vi "HOST sample code.vi"() -> ()   [LabVIEW 2020]
uses:
  <vilib>/Platform/TimedLoop/XDataNode/timing_clust.ctl
  <vilib>/Platform/TimedLoop/XDataNode/nitl_modes.ctl
  <vilib>/Platform/TimedLoop/XDataNode/wakeup.ctl
  <vilib>/Platform/TimedLoop/XDataNode/XDataNode.xnode
  <vilib>/Platform/TimedLoop/XDataNode/XDNodeRunTimeDep.lvlib
panel:
  out "Status word":u16
  in  "Sine test":bool caption="空白按钮"
  in  "Message ID":u32
  in  "descend":bool caption="空白按钮"
  in  "run":bool caption="空白按钮"
  in  "neutral":bool caption="空白按钮"
  in  "host ip":string="127.0.0.1"
  in  "base ip":string="127.0.0.1"
  in  "Command word":u16
  out "sway/surge/heave":T1(graph)
  out "pitch/roll/yaw":T2(graph)
  out "Stroke1..6":T3(graph)
  out "DataToHOST":T4 {"actuator6_pos" format="%#.2f"; "actuator5_pos" format="%#.2f"; "actuator4_pos" format="%#.2f"; "actuator3_pos" format="%#.2f"; "actuator2_pos" format="%#.2f"; "actuator1_pos" format="%#.2f"; "driver6 torque" format="%#.2f"; "driver5 torque" format="%#.2f"; "driver4 torque" format="%#.2f"; "driver3 torque" format="%#.2f"; "driver2 torque" format="%#.2f"; "driver1 torque" format="%#.2f"; "errorCode6(hex)" format="%x"; "errorCode5(hex)" format="%x"; "errorCode4(hex)" format="%x"; "errorCode3(hex)" format="%x"; "errorCode2(hex)" format="%x"; "errorCode1(hex)" format="%x"; "Heave actual" format="%#.2f"; "Surge actual" format="%#.2f"; "Sway actual" format="%#.2f"; "Yaw actual" format="%#.2f"; "Roll actual" format="%#.2f"; "Pitch actual" format="%#.2f"; "IO word" format="%x"}
  in  "host port":u16=10010
  in  "base port":u16=10000
  out "DataToDOF":T5={"Packet lenght"=48, "sequence count"=0, "Reserved"=0, "Message ID"=0, "Command word"=0, "Playback file ID"=0, "SubCmd"=0, "Reserved3"=0, "Reserved4"=0, "Reserved5"=0, "PITCH"=0.0, "ROLL"=0.0, "YAW"=0.0, "SWAY"=0.0, "SURGE"=0.0, "HEAVE"=0.0, "var11"=0.0, "var12"=0.0, "var13"=0.0, "var14"=0.0, "var15"=0.0, "var16"=0.0, "var21"=0.0, "var22"=0.0, "var23"=0.0, "var24"=0.0, "var25"=0.0, "var26"=0.0, "var31"=0.0, "var32"=0.0, "var33"=0.0, "var34"=0.0, "var35"=0.0, "var36"=0.0} {"Reserved5" format="%x"; "Reserved4" format="%x"; "Reserved3" format="%x"}
  in  "停止":bool
  # "概述：演示使用UDP通讯控制运动模拟器并显示其状态。\n操作步骤：\n1.网络链接运动模拟器，设置好IP和端口；\n2.运行VI，点击界面按钮，控制模拟器动作；\n3.单击停止 停止VI运行。"
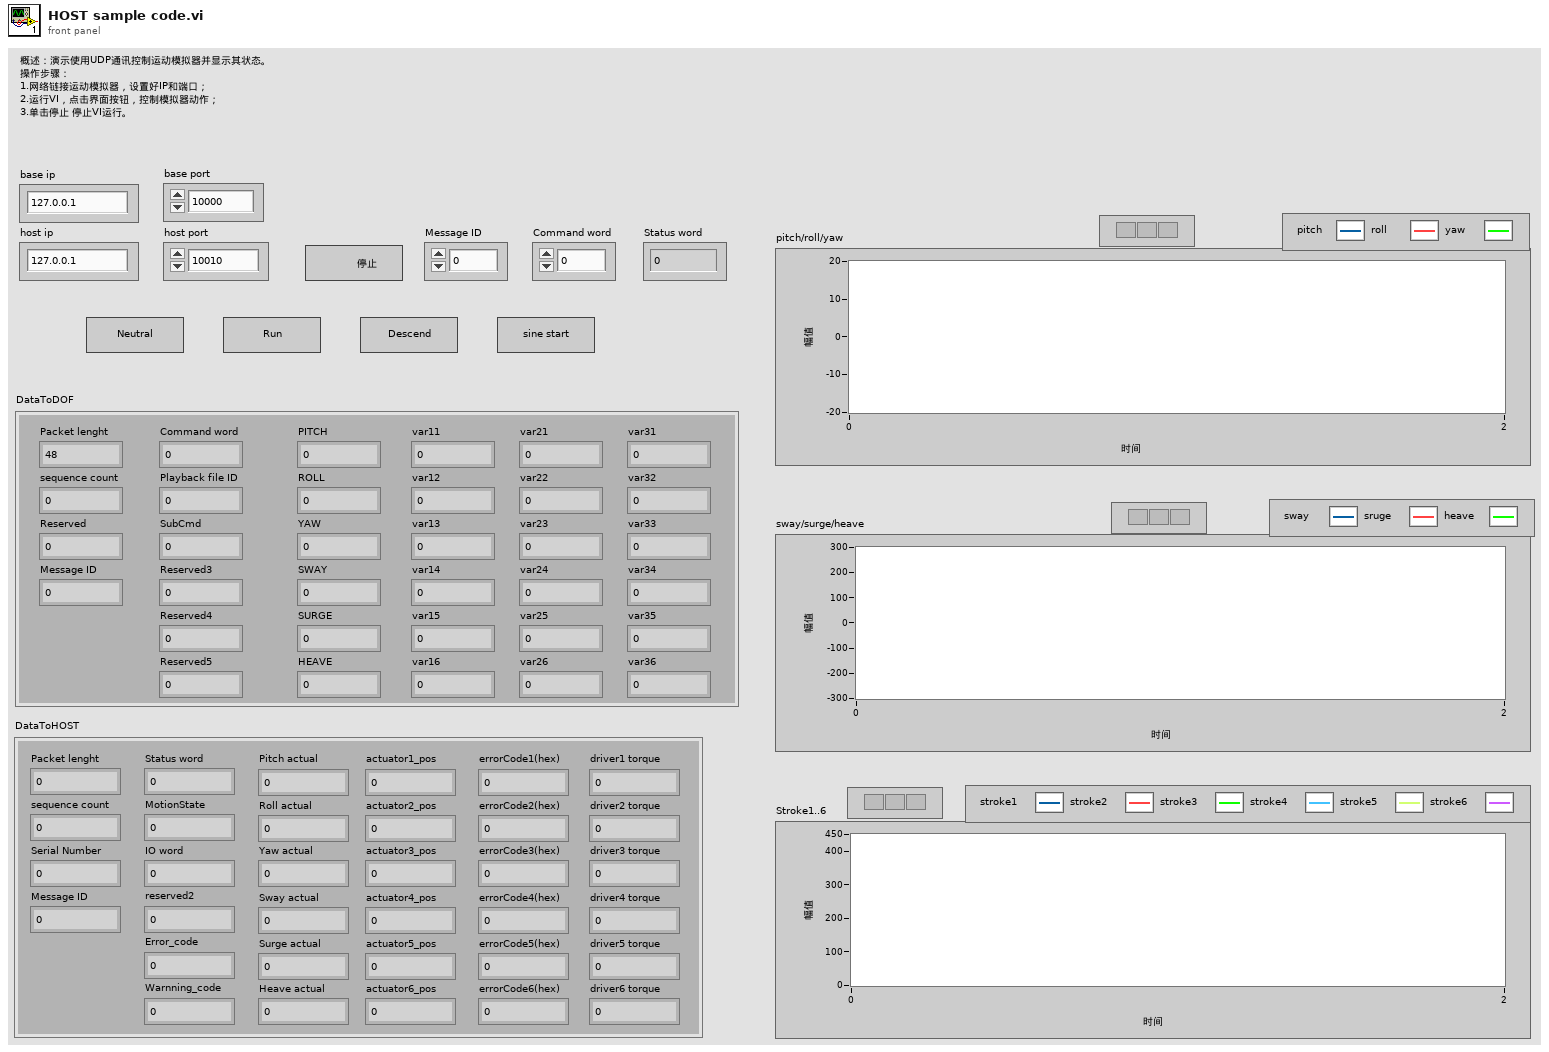
[diagram p1: front panel]
types:
  T1 = cluster{"Sway actual ":sgl, "Surge actual ":sgl, "Heave actual ":sgl}
  T2 = cluster{"Pitch actual ":sgl, "Roll actual ":sgl, "Yaw actual ":sgl}
  T3 = cluster{"actuator1_pos":sgl, "actuator2_pos":sgl, "actuator3_pos":sgl, "actuator4_pos":sgl, "actuator5_pos":sgl, "actuator6_pos":sgl}
  T4 = cluster{"Packet lenght":u32, "sequence count":u32, "Serial Number":u32, "Message ID":u32, "Status word":u16, "MotionState":u16, "IO word":u16, "reserved2":u16, "Error_code":u32, "Warnning_code":u32, "Pitch actual ":sgl, "Roll actual ":sgl, "Yaw actual ":sgl, "Sway actual ":sgl, "Surge actual ":sgl, "Heave actual ":sgl, "actuator1_pos":sgl, "actuator2_pos":sgl, "actuator3_pos":sgl, "actuator4_pos":sgl, "actuator5_pos":sgl, "actuator6_pos":sgl, "errorCode1(hex)":u32, "errorCode2(hex)":u32, "errorCode3(hex)":u32, "errorCode4(hex)":u32, "errorCode5(hex)":u32, "errorCode6(hex)":u32, "driver1 torque":sgl, "driver2 torque":sgl, "driver3 torque":sgl, "driver4 torque":sgl, "driver5 torque":sgl, "driver6 torque":sgl}
  T5 = cluster{"Packet lenght":u32, "sequence count":u32, "Reserved":u32, "Message ID":u32, "Command word":u16, "Playback file ID":u16, "SubCmd":u16, "Reserved3":u16, "Reserved4":u32, "Reserved5":u32, "PITCH":sgl, "ROLL":sgl, "YAW":sgl, "SWAY":sgl, "SURGE":sgl, "HEAVE":sgl, "var11":sgl, "var12":sgl, "var13":sgl, "var14":sgl, "var15":sgl, "var16":sgl, "var21":sgl, "var22":sgl, "var23":sgl, "var24":sgl, "var25":sgl, "var26":sgl, "var31":sgl, "var32":sgl, "var33":sgl, "var34":sgl, "var35":sgl, "var36":sgl}
  T6 = typedef "XDNodeRunTimeDep.lvlib/timing_clust.ctl" = cluster{"Expected End [f-1]":u64, "Actual End [f-1]":u64, "Finished Late? [f-1]":bool, "Expected End [i-1]":u64, "Actual End [i-1]":u64, "Finished Late? [i-1]":bool, "Expected Start [i]":u64, "Actual Start [i]":u64, "Expected Start [f]":u64, "Actual Start [f]":u64, "Source Name":string, "Structure Name":string, "Period":i64, "Deadline":i64, "Offset":i64, "Start":i64, "Priority":i32, "Timeout":i32, "Mode":T7, "Wakeup Reason":T8, "Error":errorcluster, "Source Type":string, "Secondary Source Type":string, "Global End Time":u64, "Global Start Time":u64, "Frame Duration":u64, "Iteration Duration":u64, "Assigned CPU":i32, "I/O Scan Engine Mode":u32}
  T7 = typedef "XDNodeRunTimeDep.lvlib/nitl_modes.ctl" = enum32{"No Change", "Process missed periods, maintain original phase", "Discard missed periods, maintain original phase", "Process missed periods, ignore original phase", "Discard missed periods, ignore original phase"}
  T8 = typedef "XDNodeRunTimeDep.lvlib/wakeup.ctl" = enum32{"Normal", "Aborted", "Asynchronous wakeup", "Timing source error", "Timed loop error", "Timeout"}
  T9 = cluster{"Packet lenght":u32, "sequence count":u32, "Reserved":u32, "Message ID":u32, "Status word":u16, "MotionState":u16, "IO word":u16, "reserved2":u16, "Error_code":u32, "Warnning_code":u32, "Pitch actual ":sgl, "Roll actual ":sgl, "Yaw actual ":sgl, "Sway actual ":sgl, "Surge actual ":sgl, "Heave actual ":sgl, "actuator1_pos":sgl, "actuator2_pos":sgl, "actuator3_pos":sgl, "actuator4_pos":sgl, "actuator5_pos":sgl, "actuator6_pos":sgl, "errorCode1":u32, "errorCode2":u32, "errorCode3":u32, "errorCode4":u32, "errorCode5":u32, "errorCode6":u32, "driver1 torque":sgl, "driver2 torque":sgl, "driver3 torque":sgl, "driver4 torque":sgl, "driver5 torque":sgl, "driver6 torque":sgl}
  T10 = enum16{"big-endian, network order", "native, host order", "little-endian"}
  T11 = cluster{"Packet lenght":u32, "sequence count":u32, "Reserved":u32, "Message ID":u32, "Command word":u16, "Playback file ID":u16, "Rserved2":u16, "Reserved3":u16, "Reserved4":u32, "Reserved5":u32, "PITCH":sgl, "ROLL":sgl, "YAW":sgl, "SWAY":sgl, "SURGE":sgl, "HEAVE":sgl, "var11":sgl, "var12":sgl, "var13":sgl, "var14":sgl, "var15":sgl, "var16":sgl, "var21":sgl, "var22":sgl, "var23":sgl, "var24":sgl, "var25":sgl, "var26":sgl, "var31":sgl, "var32":sgl, "var33":sgl, "var34":sgl, "var35":sgl, "var36":sgl}
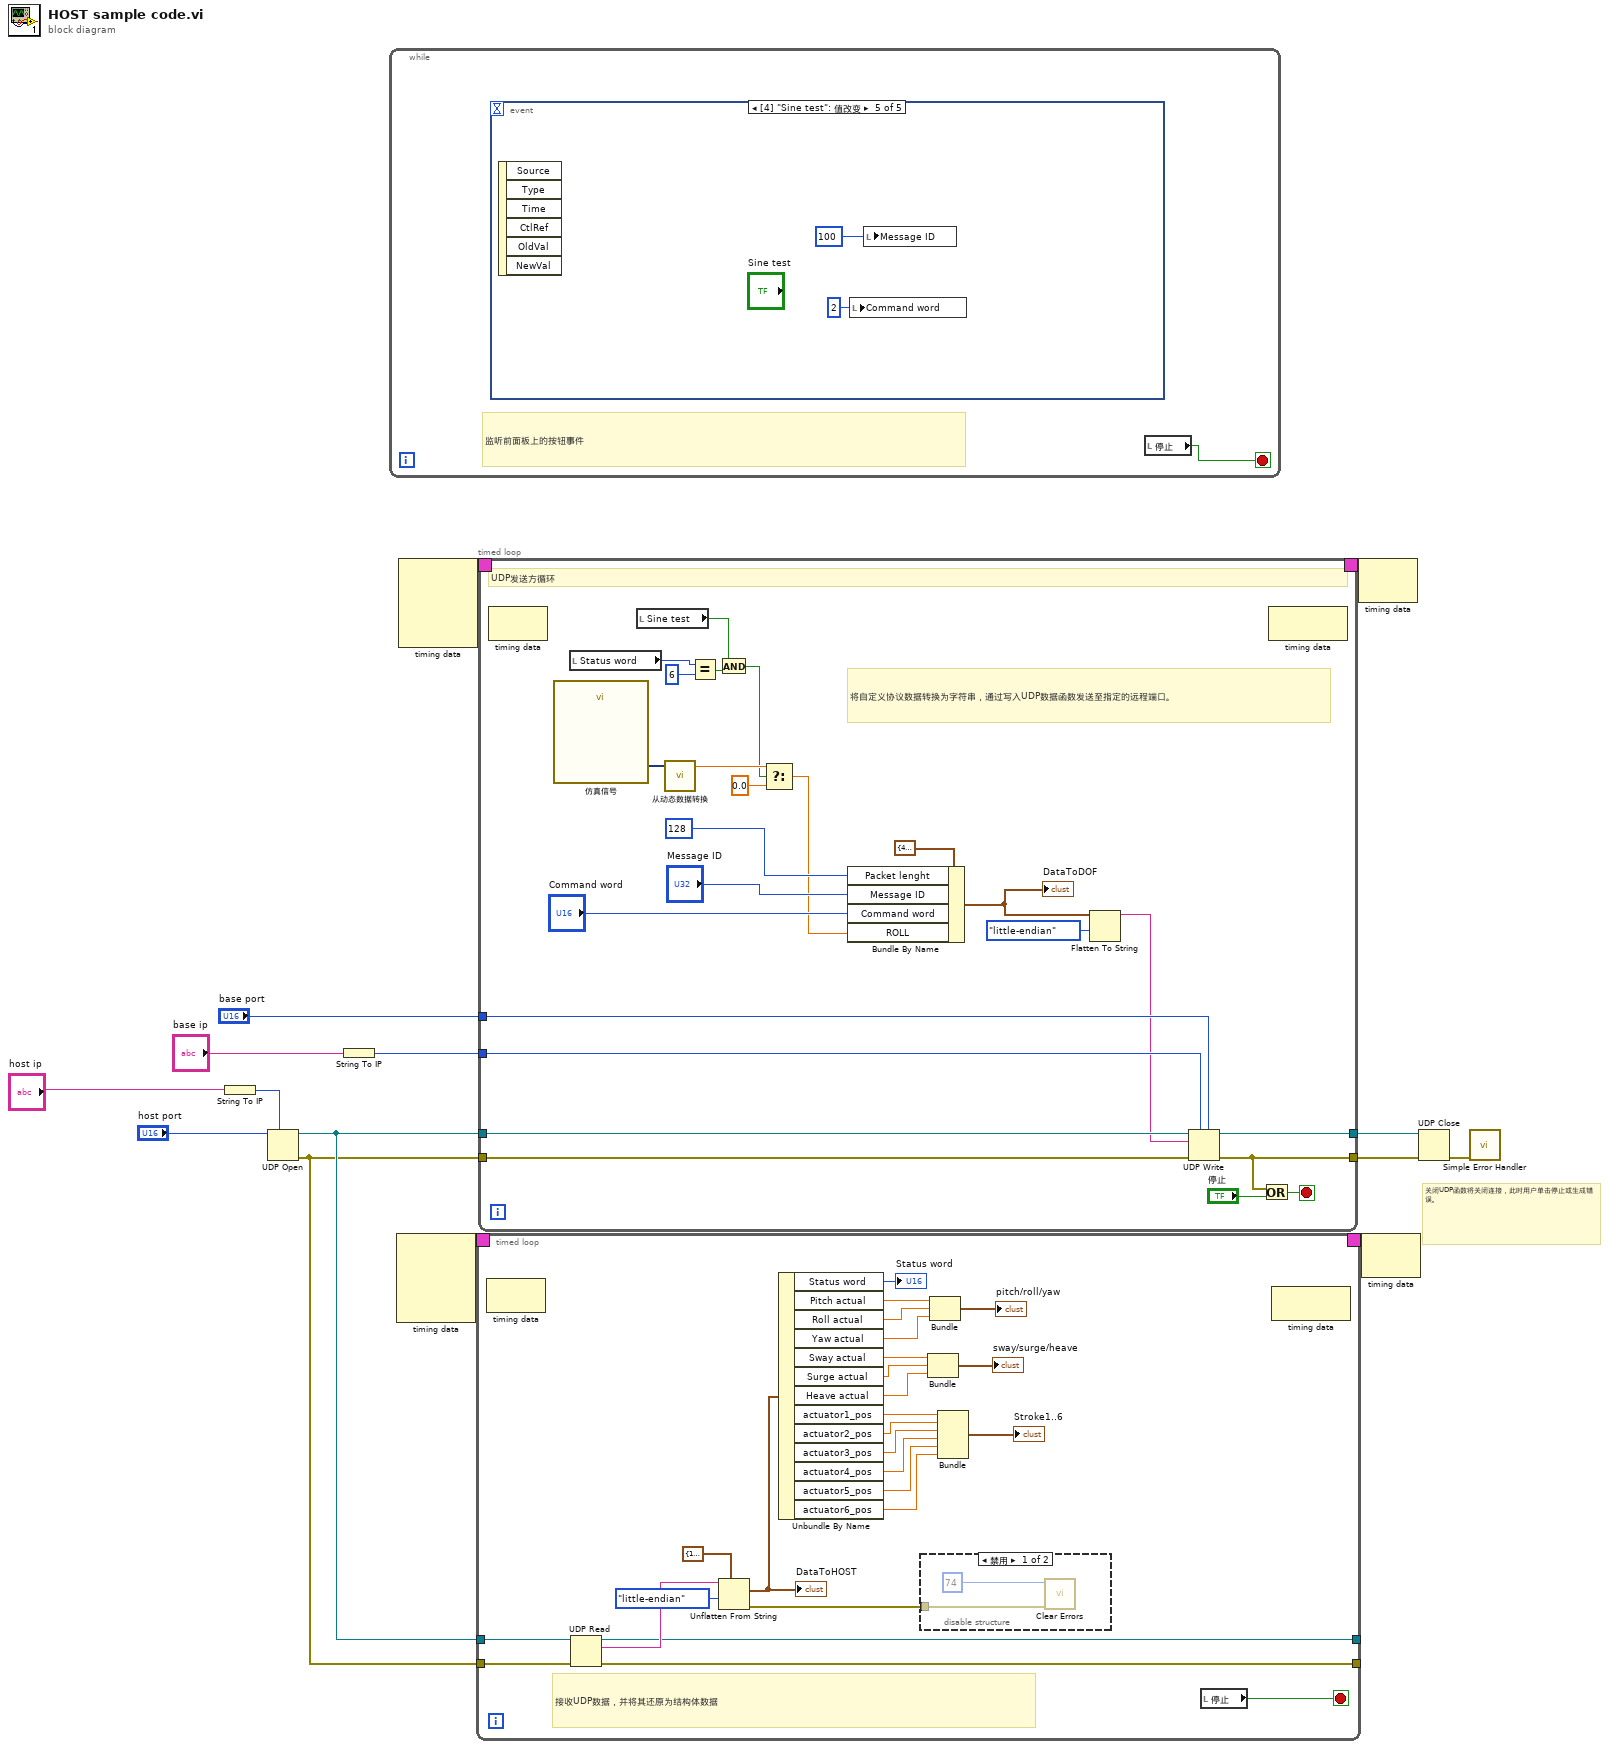
[diagram p0: block diagram]
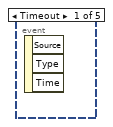
[diagram p2: hidden frame]
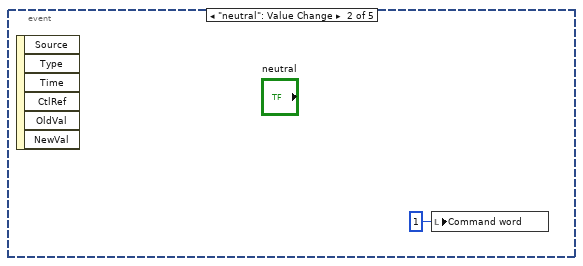
[diagram p3: hidden frame]
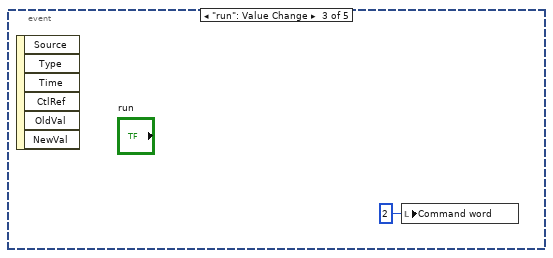
[diagram p4: hidden frame]
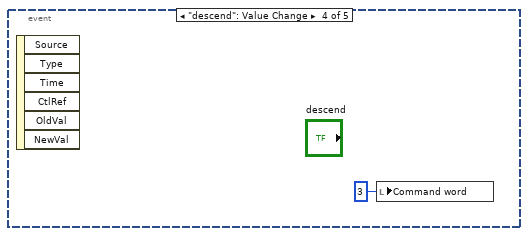
[diagram p5: hidden frame]
diagram:
  # "关闭UDP函数将关闭连接，此时用户单击停止或生成错误。"
  n1 = String To IP(1:"host ip") -> (0:w7:u32)
  n2 = UDP Open(7:w7, 11:"host port") -> (port=w6:refnum<k16>, 0:w5:errorcluster)  [unwired: 3 in, 1 out]
  n3 = String To IP(1:"base ip") -> (0:w12:u32)
  n4 = while {
    stop <- w16 stop-if-true
    # "监听前面板上的按钮事件"
    n5 = event shown="[4] \"Sine test\": 值改变" {
      selector: _ -> [_ _ _ _ _]
      dyn-events: _ -> [_ _ _ _ _]
      timeout: _ -> [_ _ _ _ _]
      event Timeout {
        n6 = event-data() -> ()  [unwired: 1 in, 3 out]
      }
      event "neutral": Value Change {
        n7 = event-data() -> ()  [unwired: 1 in, 6 out]
        n8 = local write "Command word"(u16 1 ("Command word")) -> ()
      }
      event "run": Value Change {
        n9 = event-data() -> ()  [unwired: 1 in, 6 out]
        n10 = local write "Command word"(u16 2 ("Command word")) -> ()
      }
      event "descend": Value Change {
        n11 = event-data() -> ()  [unwired: 1 in, 6 out]
        n12 = local write "Command word"(u16 3 ("Command word")) -> ()
      }
      event "Sine test": Value Change {
        n13 = event-data() -> ()  [unwired: 1 in, 6 out]
        n14 = local write "Command word"(u16 2 ("Command word")) -> ()
        n15 = local write "Message ID"(u32 100 ("Command word")) -> ()
      }
    }
    n16 = local read "停止"() -> (w16:bool)
  }
  n17 = node-c288() -> (w4:T6)  [unwired: 4 in]
  n18 = node-c288() -> (w9:T6)  [unwired: 4 in]
  n19 = timed-loop {
    timing: w4 -> [_]
    timing-out: [_] -> w3
    tunnel: w6 -> [w47]
    tunnel: w5 -> [w46]
    tunnel: [w43] -> _
    tunnel: [w42] -> _
    stop <- w39 stop-if-true
    # "接收UDP数据，并将其还原为结构体数据"
    n20 = node-c288() -> ()  [unwired: 1 in, 1 out]
    n21 = UDP Read(connection ID=w47, 8:w46) -> (data out=w45:string, error out=w42:errorcluster, 3:w43:refnum<k16>)  [unwired: 2 in, 2 out]
    n22 = Unflatten From String(type=T9 {"Packet lenght"=128, "sequence count"=0, "Reserved"=0, "Message ID"=0, "Status word"=16, "MotionState"=257, "IO word"=0, "reserved2"=0, "Error_code"=0, "Warnning_code"=0, "Pitch actual "=0.0, "Roll actual "=0.0, "Yaw actual "=0.0, "Sway actual "=0.0, "Surge actual "=0.0, "Heave actual "=0.0, "actuator1_pos"=0.0, "actuator2_pos"=0.0, "actuator3_pos"=0.0, "actuator4_pos"=0.0, "actuator5_pos"=0.0, "actuator6_pos"=0.0, "errorCode1"=0, "errorCode2"=0, "errorCode3"=0, "errorCode4"=0, "errorCode5"=0, "errorCode6"=0, "driver1 torque"=0.0, "driver2 torque"=0.0, "driver3 torque"=0.0, "driver4 torque"=0.0, "driver5 torque"=0.0, "driver6 torque"=0.0} ("DataToHOST 2"), binary string=w45, byte order (0:big-endian, network order)=T10."little-endian" ("字节顺序(0:big-endian, network order)")) -> (value=w40:T9, error out=w41:errorcluster)  [unwired: 2 in, 1 out]
    "DataToHOST" <- w40
    n23 = Unbundle By Name(w40) -> ("Status word"=→"Status word":u16, "Pitch actual"=w37:sgl, "Roll actual"=w36:sgl, "Yaw actual"=w35:sgl, "Sway actual"=w33:sgl, "Surge actual"=w32:sgl, "Heave actual"=w31:sgl, "actuator1_pos"=w29:sgl, "actuator2_pos"=w28:sgl, "actuator3_pos"=w27:sgl, "actuator4_pos"=w26:sgl, "actuator5_pos"=w25:sgl, "actuator6_pos"=w24:sgl)
    n24 = disable-structure shown="禁用" {
      disable-tunnel: w41 -> [w49 _]
      frame Disabled {
        n25 = call <vilib>:"Clear Errors.vi"("error in (no error)"=w49, "specific error code to clear (0: all)"=74 ("error code (no error:0)")) -> ()  [unwired: 4 in, 2 out]
      }
      frame Enabled {
      }
    }
    n26 = Bundle("Sway actual"=w33, "Surge actual"=w32, "Heave actual"=w31) -> (→"sway/surge/heave":T1)  [unwired: 1 in]
    n27 = Bundle("Pitch actual"=w37, "Roll actual"=w36, "Yaw actual"=w35) -> (→"pitch/roll/yaw":T2)  [unwired: 1 in]
    n28 = Bundle("actuator1_pos"=w29, "actuator2_pos"=w28, "actuator3_pos"=w27, "actuator4_pos"=w26, "actuator5_pos"=w25, "actuator6_pos"=w24) -> (→"Stroke1..6":T3)  [unwired: 1 in]
    n29 = local read "停止"() -> (w39:bool)
    n30 = node-c288() -> ()  [unwired: 1 in, 1 out]
  }
  n31 = timed-loop {
    tunnel: [w75] -> w14
    tunnel: w6 -> [w74]
    tunnel: w5 -> [w73]
    tunnel: [w72] -> w15
    tunnel: w12 -> [w71]
    tunnel: "base port" -> [w70]
    timing: w9 -> [_]
    timing-out: [_] -> w8
    stop <- w69 stop-if-true
    # "将自定义协议数据转换为字符串，通过写入UDP数据函数发送至指定的远程端口。"
    # "UDP发送方循环"
    n32 = node-c288() -> ()  [unwired: 1 in, 1 out]
    n33 = call "仿真信号"() -> ("正弦"=w64:dynamicdata)  [unwired: 14 in, 1 out]
    n34 = local read "Status word"() -> (w56:u16)
    n35 = local read "Sine test"() -> (w53:bool)
    n36 = call "从动态数据转换"("Dynamic Data Type"=w64) -> ("Scalar"=w59:dbl)  [unwired: 3 in]
    n37 = Equal?(x=w56, y=u16 6) -> (x = y?=w54:bool)
    n38 = And(x=w53, y=w54) -> (x .and. y?=w52:bool)
    n39 = Select(t=w59, s=w52, f=0.0) -> (s? t:f=w57:dbl)
    n40 = Bundle By Name(cluster=T11 {"Packet lenght"=48, "sequence count"=0, "Reserved"=0, "Message ID"=0, "Command word"=0, "Playback file ID"=0, "Rserved2"=0, "Reserved3"=0, "Reserved4"=0, "Reserved5"=0, "PITCH"=0.0, "ROLL"=0.0, "YAW"=0.0, "SWAY"=0.0, "SURGE"=0.0, "HEAVE"=0.0, "var11"=0.0, "var12"=0.0, "var13"=0.0, "var14"=0.0, "var15"=0.0, "var16"=0.0, "var21"=0.0, "var22"=0.0, "var23"=0.0, "var24"=0.0, "var25"=0.0, "var26"=0.0, "var31"=0.0, "var32"=0.0, "var33"=0.0, "var34"=0.0, "var35"=0.0, "var36"=0.0} ("DataToDOF 2"), "Packet lenght"=u32 128, "Message ID"="Message ID", "Command word"="Command word", "ROLL"=w57) -> (w63:T11)
    "DataToDOF" <- w63
    n41 = Flatten To String(anything=w63, byte order (0:big-endian, network order)=T10."little-endian" ("字节顺序(0:big-endian, network order)")) -> (data string=w66:string)  [unwired: 2 in, 2 out]
    n42 = UDP Write(address=w71, port or service name=w70, connection ID=w74, data in=w66, 8:w73) -> (error out=w75:errorcluster, 3:w72:refnum<k16>)  [unwired: 1 in]
    n43 = Or(x=w75, y="停止") -> (x .or. y?=w69:bool)
    n44 = node-c288() -> ()  [unwired: 1 in, 1 out]
  }
  n45 = node-c288(w8) -> ()  [unwired: 1 out]
  n46 = node-c288(w3) -> ()  [unwired: 1 out]
  n47 = UDP Close(connection ID=w15, 8:w14) -> (error out=w13:errorcluster)  [unwired: 1 out]
  n48 = call <vilib>:"Simple Error Handler.vi"("error in (no error)"=w13) -> ()  [unwired: 4 in, 5 out]
